vi "Teleop.vi"(10 "Match Info":T1={"Autonomous Elapsed Seconds"=0.0, "TeleOp Elapsed Seconds"=0.0, "Disabled Elapsed Seconds"=0.0, "Visited Autonomous"=FALSE, "Visited TeleOp"=FALSE, "Visited Disabled"=FALSE, "Autonomous Settings"={"Autonomous Style"=enum."Independent", "VI Refnum"=refnum}}, 11 "Call Context":T2) -> ()   [LabVIEW 2014]
doc: "This VI is called for each TeleOp packet received from the DS where the robot is not disabled. It is often used to read from the joysticks and update I/O or to update setpoints for timed control loops. It should complete and return within 20 milliseconds or it may miss DS packets."
uses:
  <vilib>/Rock Robotics/WPI/DriverStation/WPI_DriverStationDerivedRobotMode.ctl
  <vilib>/Rock Robotics/WPI/DriverStation/WPI_DriverStationMatch Info.ctl
  <vilib>/Rock Robotics/WPI/DriverStation/DriverStationLCD/WPI_DriverStationLCDLCDLine.ctl
  <vilib>/Rock Robotics/WPI/Joystick/WPI_JoystickGetSetRefNum.vi
  Robot Global Data.vi
  <vilib>/Rock Robotics/WPI/RobotDrive/WPI_RobotDriveGetSetRefNum.vi
  <vilib>/Rock Robotics/WPI/RobotDrive/WPI_RobotDriveArcadeDrive_Standard(NoSaturation).vi
  <vilib>/Rock Robotics/WPI/Solenoid/Deprecated/WPI_SolenoidSetBool.vi
panel:
  out "Numeric 1":dbl(slide) scale=0.0..100.0
  out "Boolean 2":bool
  out "Boolean 1":bool
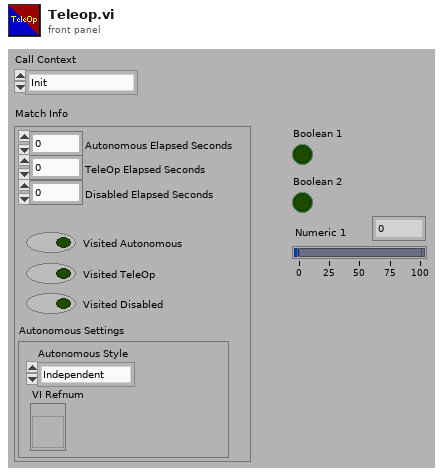
[diagram p1: front panel]
types:
  T1 = typedef "WPI_DriverStationMatch Info.ctl" = cluster{"Autonomous Elapsed Seconds":dbl, "TeleOp Elapsed Seconds":dbl, "Disabled Elapsed Seconds":dbl, "Visited Autonomous":bool, "Visited TeleOp":bool, "Visited Disabled":bool, "Autonomous Settings":cluster{"Autonomous Style":enum16{"Iterative", "Independent"}, "VI Refnum":refnum<vi>}}
  T2 = typedef "WPI_DriverStationDerivedRobotMode.ctl" = enum16{"Init", "Execute", "Stop"}
  T3 = typedef "WPI_DriverStationLCDLCDLine.ctl" = enum16{"Main - Line 1", "User - Line 2", "User - Line 3", "User - Line 4", "User - Line 5", "User - Line 6"}
  T4 = typedef "WPI_DigitalInputDevRef.ctl" = cluster{"DevStatus":errorcluster, "DIO Channel":T5, "Digital Module":T6}
  T5 = typedef "FPGA_DIOChannel.ctl" = enum8{"DIO 1", "DIO 2", "DIO 3", "DIO 4", "DIO 5", "DIO 6", "DIO 7", "DIO 8", "DIO 9", "DIO 10", "DIO 11", "DIO 12", "DIO 13", "DIO 14", "Invalid"}
  T6 = typedef "FPGA_TypedefDigitalModule.ctl" = enum16{"Digital Module 1", "Digital Module 2"}
  T7 = typedef "WPI_JoystickDevRef.ctl" = cluster{"Device":T8}
  T8 = typedef "WPI_JoystickDeviceEnum.ctl" = enum16{"USB 0", "USB 1", "USB 2", "USB 3", "USB 4", "USB 5"}
  T9 = cluster{"Button 1":bool, "Button 2":bool, "Button 3":bool, "Button 4":bool, "Button 5":bool, "Button 6":bool, "Button 7":bool, "Button 8":bool, "Button 9":bool, "Button 10":bool, "Button 11":bool, "Button 12":bool}
  T10 = cluster{"axis 1 (x)":dbl, "axis 2 (y)":dbl, "axis 3 (throttle)":dbl, "axis 4":dbl, "axis 5":dbl, "axis 6":dbl}
  T11 = typedef "WPI_MotorControlDeviceRef.ctl" = cluster{"DeviceStatus":errorcluster, "Type":enum16{"PWM", "CAN"}, "PWM":cluster{"Digital Module":T6, "PWM Channel":T12, "DeadBand":T13}, "CAN":cluster{"Device Number":u8, "Control Mode":T14, "Semaphore":T15, "Max Vout":dbl}, "Invert":bool, "TransformRef":T16, "InvTransformRef":T16}
  T12 = typedef "FPGA_DIOPWMChannel.ctl" = enum8{"PWM 1", "PWM 2", "PWM 3", "PWM 4", "PWM 5", "PWM 6", "PWM 7", "PWM 8", "PWM 9", "PWM 10", "Invalid"}
  T13 = typedef "WPI_PWMDeadband.ctl" = cluster{"Name":string, "maxPositivePwm":i32, "minPositivePwm":i32, "centerPwm":i32, "maxNegativePwm":i32, "minNegativePwm":i32, "angularRange":u16}
  T14 = typedef "WPI_CANJaguar_ControlMode.ctl" = enum8{"Percent VBus", "Current", "Speed", "Position", "Voltage"}
  T15 = typedef "Semaphore RefNum" = refnum<k1>
  T16 = typedef "WPI_PWMTransform_ConPane.ctl" = refnum<vi>
  T17 = typedef "WPI_SolenoidDevRef.ctl" = cluster{"DevStatus":errorcluster, "Solenoid Module":T18, "Forward Solenoid Channel":T19, "Reverse Solenoid Channel":T19}
  T18 = typedef "FPGA_TypedefSolenoidModule.ctl" = enum16{"Solenoid Module 1", "Solenoid Module 2"}
  T19 = typedef "WPI_SolenoidChannel.ctl" = enum8{"Solenoid 1", "Solenoid 2", "Solenoid 3", "Solenoid 4", "Solenoid 5", "Solenoid 6", "Solenoid 7", "Solenoid 8", "Invalid"}
  T20 = typedef "WPI_RobotDriveDevRef.ctl" = cluster{"DevStatus":errorcluster, "Motors[]":T11[], "Square Inputs":bool, "Max Output":dbl}
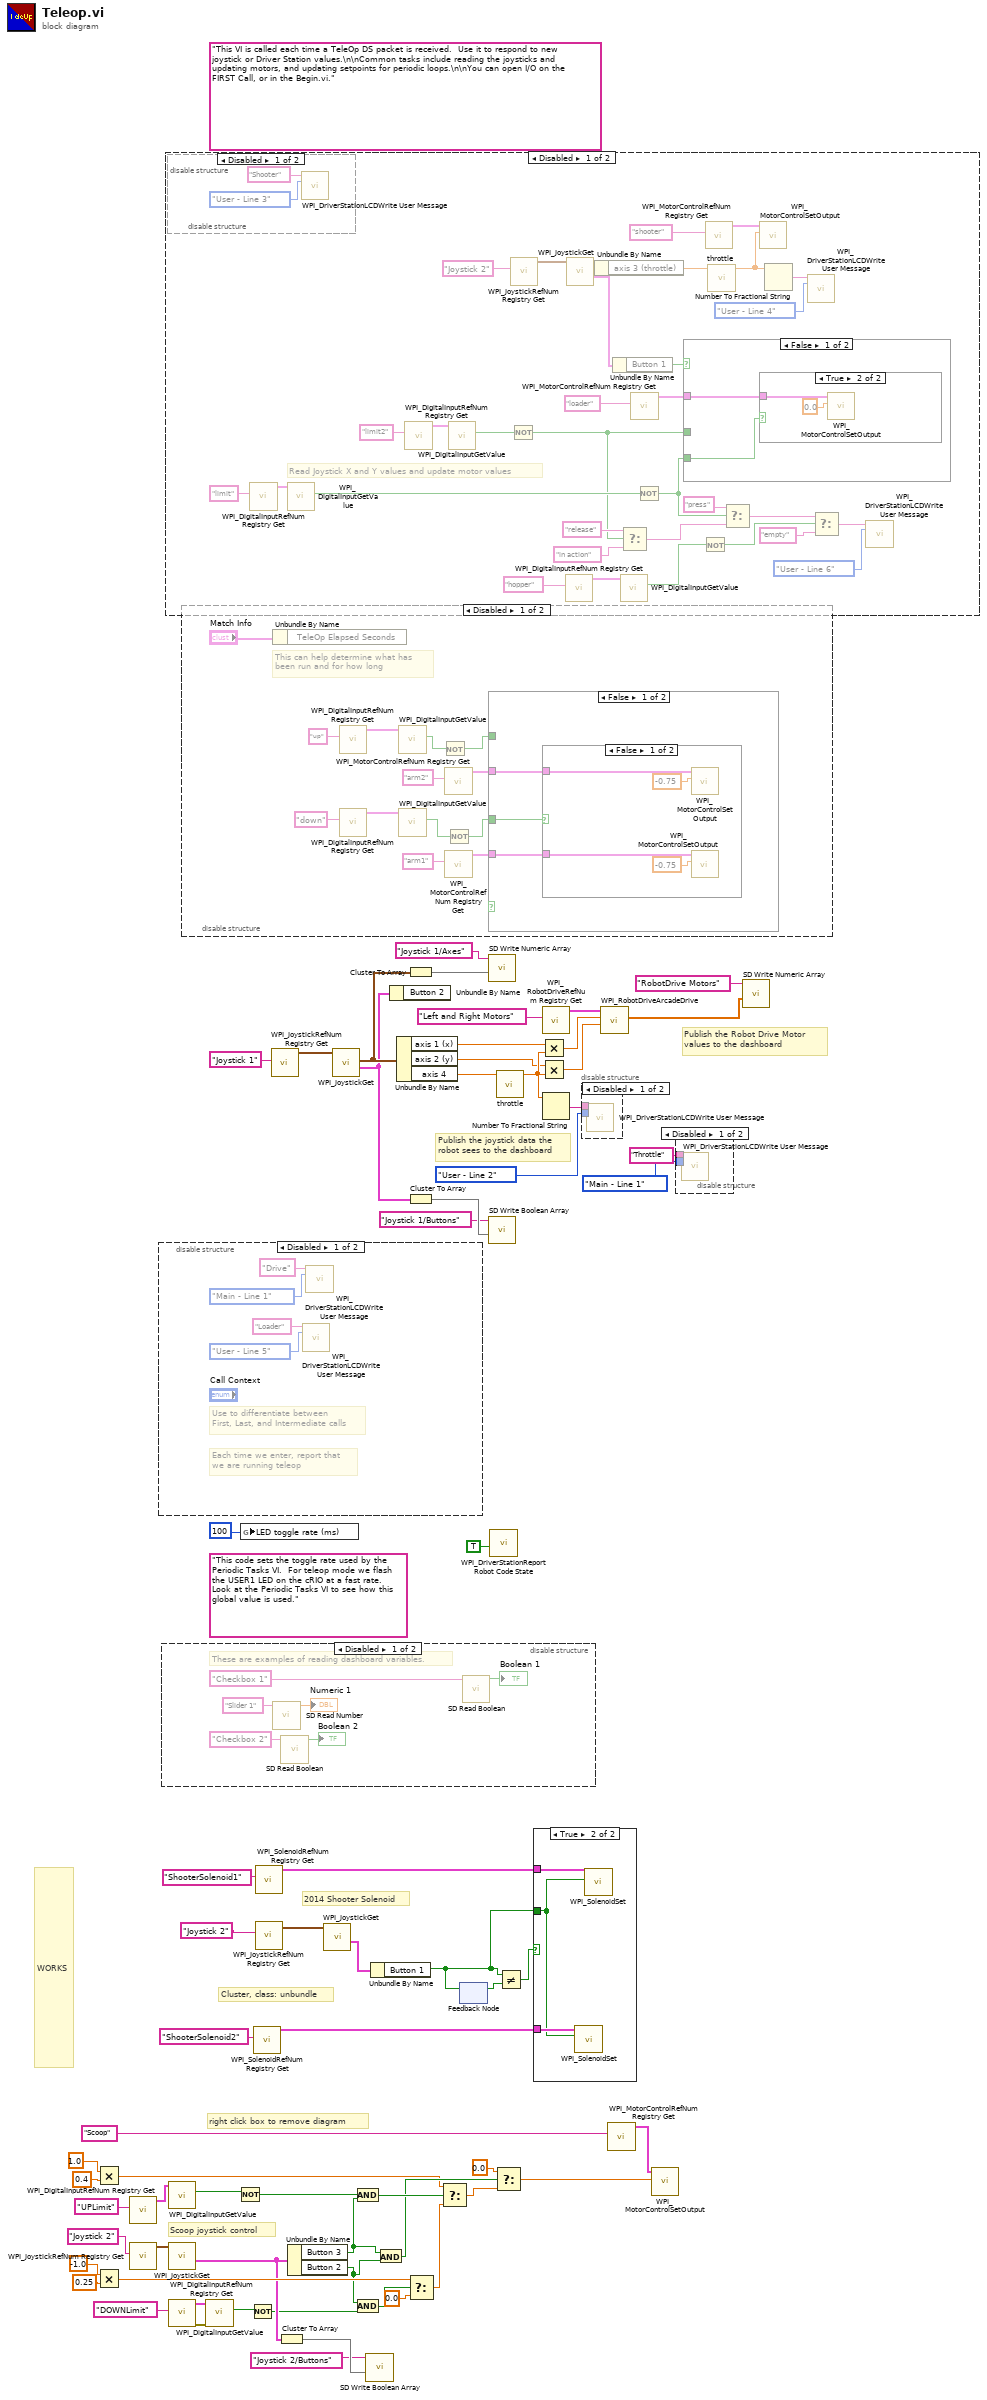
[diagram p0: block diagram]
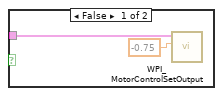
[diagram p4: hidden frame]
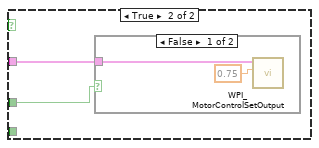
[diagram p5: hidden frame]
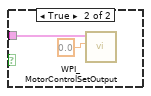
[diagram p6: hidden frame]
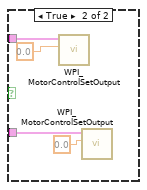
[diagram p12: hidden frame]
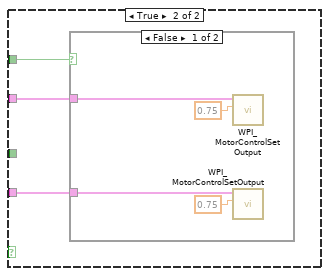
[diagram p13: hidden frame]
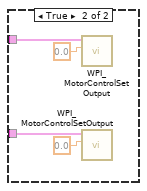
[diagram p14: hidden frame]
diagram:
  (unwired) "This code sets the toggle rate used by the Periodic Tasks VI.  For teleop mode we flash the USER1 LED on the cRIO at a fast rate.  Look at the Periodic Tasks VI to see how this global value is used."
  (unwired) "This VI is called each time a TeleOp DS packet is received.  Use it to respond to new joystick or Driver Station values.\n\nCommon tasks include reading the joysticks and updating motors, and updating setpoints for periodic loops.\n\nYou can open I/O on the FIRST Call, or in the Begin.vi."
  # "right click box to remove diagram"
  # "Scoop joystick control"
  # "WORKS"
  # "2014 Shooter Solenoid"
  # "Cluster, class: unbundle"
  # "Publish the Robot Drive Motor\nvalues to the dashboard"
  # "Publish the joystick data the\nrobot sees to the dashboard"
  n1 = Multiply(x=1.0, y=0.4) -> (x*y=w14:dbl)
  n2 = Multiply(x=-1.0, y=0.25) -> (x*y=w15:dbl)
  n3 = call <vilib>:"WPI_DigitalInputRefNum Registry Get.vi"("refnum name"="UPLimit") -> ("DigitalInputDevRef"=w29:T4)  [unwired: 9 in, 1 out]
  n4 = call <vilib>:"WPI_JoystickRefNum Registry Get.vi"("refnum name"="Joystick 2") -> ("JoystickDevRef"=w32:T7)  [unwired: 9 in, 1 out]
  n5 = disable-structure shown="Disabled" {
    frame Disabled {
      # "Each time we enter, report that\nwe are running teleop"
      # "Use to differentiate between\nFirst, Last, and Intermediate calls"
      n6 = call <vilib>:"WPI_DriverStationLCDWrite User Message.vi"("line text"="Loader", "line"=WPI_DriverStationLCDLCDLine."User - Line 5") -> ()  [unwired: 13 in, 1 out]
      n7 = call <vilib>:"WPI_DriverStationLCDWrite User Message.vi"("line text"="Drive", "line"=WPI_DriverStationLCDLCDLine."Main - Line 1") -> ()  [unwired: 13 in, 1 out]
    }
    frame Enabled {
    }
  }
  n8 = disable-structure shown="Disabled" {
    frame Disabled {
      # "These are examples of reading dashboard variables."
      n9 = call <vilib>:"SD Read Number.vi"("Name"="Slider 1" ("refnum name")) -> ("Numeric"=→"Numeric 1":dbl)  [unwired: 8 in, 2 out]
      n10 = call <vilib>:"SD Read Boolean.vi"("Name"="Checkbox 2" ("refnum name")) -> ("Boolean"=→"Boolean 2":bool)  [unwired: 8 in, 2 out]
      n11 = call <vilib>:"SD Read Boolean.vi"("Name"="Checkbox 1" ("refnum name")) -> ("Boolean"=→"Boolean 1":bool)  [unwired: 8 in, 2 out]
    }
    frame Enabled {
    }
  }
  n12 = disable-structure shown="Disabled" {
    frame Disabled {
      # "Read Joystick X and Y values and update motor values"
      n13 = disable-structure shown="Disabled" {
        frame Disabled {
          n14 = call <vilib>:"WPI_DriverStationLCDWrite User Message.vi"("line text"="Shooter", "line"=WPI_DriverStationLCDLCDLine."User - Line 3") -> ()  [unwired: 13 in, 1 out]
        }
        frame Enabled {
        }
      }
      n15 = call <vilib>:"WPI_DigitalInputRefNum Registry Get.vi"("refnum name"="limit") -> ("DigitalInputDevRef"=w106:T4)  [unwired: 9 in, 1 out]
      n16 = call <vilib>:"WPI_DigitalInputGetValue.vi"("DigitalInputDevRef"=w106) -> ("Value"=w100:bool)  [unwired: 8 in, 2 out]
      n17 = call <vilib>:"WPI_DigitalInputRefNum Registry Get.vi"("refnum name"="limit2") -> ("DigitalInputDevRef"=w102:T4)  [unwired: 9 in, 1 out]
      n18 = call <vilib>:"WPI_DigitalInputGetValue.vi"("DigitalInputDevRef"=w102) -> ("Value"=w101:bool)  [unwired: 8 in, 2 out]
      n19 = Not(x=w101) -> (.not. x?=w94:bool)
      n20 = call <vilib>:"WPI_JoystickRefNum Registry Get.vi"("refnum name"="Joystick 2") -> ("JoystickDevRef"=w92:T7)  [unwired: 1 in, 9 out]
      n21 = call <vilib>:"WPI_DigitalInputRefNum Registry Get.vi"("refnum name"="hopper") -> ("DigitalInputDevRef"=w82:T4)  [unwired: 9 in, 1 out]
      n22 = call <vilib>:"WPI_JoystickGet.vi"("JoystickDevRef"=w92) -> ("Buttons"=w89:T9, "Axes"=w90:T10)  [unwired: 1 in, 4 out]
      n23 = Unbundle By Name(w90) -> ("axis 3 (throttle)"=w88:dbl)
      n24 = Unbundle By Name(w89) -> ("Button 1"=w85:bool)
      n25 = call <vilib>:"WPI_DigitalInputGetValue.vi"("DigitalInputDevRef"=w82) -> ("Value"=w81:bool)  [unwired: 8 in, 2 out]
      n26 = Select(t="release", s=w94, f="in action") -> (s? t:f=w99:string)
      n27 = call <vilib>:"WPI_MotorControlRefNum Registry Get.vi"("refnum name"="loader") -> ("MotorControlDevRef"=w93:T11)  [unwired: 9 in, 1 out]
      n28 = Not(x=w100) -> (.not. x?=w95:bool)
      n29 = case shown="False" w85 {
        tunnel: w93 -> [w110 w116]
        tunnel: w94 -> [_ w117]
        tunnel: w95 -> [w111 _]
        frame False {
          n30 = case shown="True" w111 {
            tunnel: w110 -> [w112 w114]
            frame False {
              n31 = call <vilib>:"WPI_MotorControlSetOutput.vi"("Output"=-0.75, "MotorControlDevRef"=w112) -> ()  [unwired: 7 in, 3 out]
            }
            frame True {
              n32 = call <vilib>:"WPI_MotorControlSetOutput.vi"("Output"=0.0, "MotorControlDevRef"=w114) -> ()  [unwired: 7 in, 3 out]
            }
          }
        }
        frame True {
          n33 = case shown="False" w117 {
            tunnel: w116 -> [w119 w121]
            frame False {
              n34 = call <vilib>:"WPI_MotorControlSetOutput.vi"("Output"=0.75, "MotorControlDevRef"=w119) -> ()  [unwired: 7 in, 3 out]
            }
            frame True {
              n35 = call <vilib>:"WPI_MotorControlSetOutput.vi"("Output"=0.0, "MotorControlDevRef"=w121) -> ()  [unwired: 7 in, 3 out]
            }
          }
        }
      }
      n36 = Not(x=w81) -> (.not. x?=w78:bool)
      n37 = call <vilib>:"WPI_MotorControlRefNum Registry Get.vi"("refnum name"="shooter") -> ("MotorControlDevRef"=w109:T11)  [unwired: 9 in, 1 out]
      n38 = call "throttle.vi"("x"=w88) -> ("x/y"=w84:dbl)  [unwired: 10 in]
      n39 = Select(t="press", s=w95, f=w99) -> (s? t:f=w80:string)
      n40 = call <vilib>:"WPI_MotorControlSetOutput.vi"("Output"=w84, "MotorControlDevRef"=w109) -> ()  [unwired: 7 in, 3 out]
      n41 = Number To Fractional String(number=w84) -> (F-format string=w87:string)  [unwired: 3 in]
      n42 = call <vilib>:"WPI_DriverStationLCDWrite User Message.vi"("line text"=w87, "line"=WPI_DriverStationLCDLCDLine."User - Line 4") -> ()  [unwired: 13 in, 1 out]
      n43 = Select(t=w80, s=w78, f="empty") -> (s? t:f=w79:string)
      n44 = call <vilib>:"WPI_DriverStationLCDWrite User Message.vi"("line text"=w79, "line"=WPI_DriverStationLCDLCDLine."User - Line 6") -> ()  [unwired: 13 in, 1 out]
    }
    frame Enabled {
    }
  }
  n45 = call <vilib>:"WPI_DigitalInputGetValue.vi"("DigitalInputDevRef"=w29) -> ("Value"=w5:bool)  [unwired: 8 in, 2 out]
  n46 = call <vilib>:"WPI_JoystickGet.vi"("JoystickDevRef"=w32) -> ("Buttons"=w8:T9)  [unwired: 4 in, 2 out]
  n47 = call <vilib>:"WPI_DigitalInputRefNum Registry Get.vi"("refnum name"="DOWNLimit") -> ("error out"=w31:errorcluster, "DigitalInputDevRef"=w30:T4)  [unwired: 9 in]
  n48 = disable-structure shown="Disabled" {
    frame Disabled {
      # "This can help determine what has\nbeen run and for how long"
      n49 = Unbundle By Name("Match Info") -> ()  [unwired: 1 out]
      n50 = call <vilib>:"WPI_DigitalInputRefNum Registry Get.vi"("refnum name"="up") -> ("DigitalInputDevRef"=w135:T4)  [unwired: 9 in, 1 out]
      n51 = call <vilib>:"WPI_DigitalInputRefNum Registry Get.vi"("refnum name"="down") -> ("DigitalInputDevRef"=w134:T4)  [unwired: 9 in, 1 out]
      n52 = call <vilib>:"WPI_DigitalInputGetValue.vi"("DigitalInputDevRef"=w135) -> ("Value"=w127:bool)  [unwired: 8 in, 2 out]
      n53 = call <vilib>:"WPI_DigitalInputGetValue.vi"("DigitalInputDevRef"=w134) -> ("Value"=w125:bool)  [unwired: 8 in, 2 out]
      n54 = Not(x=w127) -> (.not. x?=w126:bool)
      n55 = call <vilib>:"WPI_MotorControlRefNum Registry Get.vi"("refnum name"="arm2") -> ("MotorControlDevRef"=w130:T11)  [unwired: 9 in, 1 out]
      n56 = call <vilib>:"WPI_MotorControlRefNum Registry Get.vi"("refnum name"="arm1") -> ("MotorControlDevRef"=w131:T11)  [unwired: 9 in, 1 out]
      n57 = Not(x=w125) -> (.not. x?=w124:bool)
      n58 = case shown="False" {
        selector: _ -> [_ _]
        tunnel: w126 -> [_ w150]
        tunnel: w124 -> [w139 _]
        tunnel: w131 -> [w138 w149]
        tunnel: w130 -> [w137 w148]
        frame False {
          n59 = case shown="False" w139 {
            tunnel: w138 -> [w141 w146]
            tunnel: w137 -> [w140 w145]
            frame False {
              n60 = call <vilib>:"WPI_MotorControlSetOutput.vi"("Output"=-0.75, "MotorControlDevRef"=w140) -> ()  [unwired: 7 in, 3 out]
              n61 = call <vilib>:"WPI_MotorControlSetOutput.vi"("Output"=-0.75, "MotorControlDevRef"=w141) -> ()  [unwired: 7 in, 3 out]
            }
            frame True {
              n62 = call <vilib>:"WPI_MotorControlSetOutput.vi"("Output"=0.0, "MotorControlDevRef"=w145) -> ()  [unwired: 7 in, 3 out]
              n63 = call <vilib>:"WPI_MotorControlSetOutput.vi"("Output"=0.0, "MotorControlDevRef"=w146) -> ()  [unwired: 7 in, 3 out]
            }
          }
        }
        frame True {
          n64 = case shown="False" w150 {
            tunnel: w149 -> [w152 w156]
            tunnel: w148 -> [w151 w155]
            frame False {
              n65 = call <vilib>:"WPI_MotorControlSetOutput.vi"("Output"=0.75, "MotorControlDevRef"=w151) -> ()  [unwired: 7 in, 3 out]
              n66 = call <vilib>:"WPI_MotorControlSetOutput.vi"("Output"=0.75, "MotorControlDevRef"=w152) -> ()  [unwired: 7 in, 3 out]
            }
            frame True {
              n67 = call <vilib>:"WPI_MotorControlSetOutput.vi"("Output"=0.0, "MotorControlDevRef"=w155) -> ()  [unwired: 7 in, 3 out]
              n68 = call <vilib>:"WPI_MotorControlSetOutput.vi"("Output"=0.0, "MotorControlDevRef"=w156) -> ()  [unwired: 7 in, 3 out]
            }
          }
        }
      }
    }
    frame Enabled {
    }
  }
  n69 = call <vilib>:"WPI_DigitalInputGetValue.vi"("error in (no error)"=w31, "DigitalInputDevRef"=w30) -> ("Value"=w7:bool)  [unwired: 7 in, 2 out]
  n70 = Not(x=w5) -> (.not. x?=w4:bool)
  n71 = global write "Robot Global Data.vi" "LED toggle rate (ms)"(u32 100 ("LED ms toggle rate")) -> ()
  n72 = Not(x=w7) -> (.not. x?=w6:bool)
  n73 = call <vilib>:"WPI_SolenoidRefNum Registry Get.vi"("refnum name"="ShooterSolenoid2") -> ("SolenoidDevRef"=w39:T17)  [unwired: 9 in, 1 out]
  n74 = call <vilib>:"WPI_SolenoidRefNum Registry Get.vi"("refnum name"="ShooterSolenoid1") -> ("SolenoidDevRef"=w44:T17)  [unwired: 9 in, 1 out]
  n75 = call <vilib>:"WPI_JoystickRefNum Registry Get.vi"("refnum name"="Joystick 2") -> ("JoystickDevRef"=w43:T7)  [unwired: 9 in, 1 out]
  n76 = call <vilib>:"WPI_JoystickRefNum Registry Get.vi"("refnum name"="Joystick 1") -> ("JoystickDevRef"=w64:T7)  [unwired: 1 in, 9 out]
  n77 = Cluster To Array(cluster=w8) -> (array=w10:bool[])
  n78 = Unbundle By Name(w8) -> ("Button 3"=w12:bool, "Button 2"=w11:bool)
  n79 = call <vilib>:"WPI_JoystickGet.vi"("JoystickDevRef"=w43) -> ("Buttons"=w41:T9)  [unwired: 4 in, 2 out]
  n80 = call <vilib>:"WPI_JoystickGet.vi"("JoystickDevRef"=w64) -> ("Buttons"=w46:T9, "Axes"=w60:T10)  [unwired: 1 in, 4 out]
  n81 = And(x=w4, y=w12) -> (x .and. y?=w26:bool)
  n82 = And(x=w11, y=w6) -> (x .and. y?=w25:bool)
  n83 = call <vilib>:"SD Write Boolean Array.vi"("Boolean Array"=w10, "Name"="Joystick 2/Buttons") -> ()  [unwired: 8 in, 2 out]
  n84 = Unbundle By Name(w41) -> ("Button 1"=w36:bool)
  n85 = And(x=w12, y=w11) -> (x .and. y?=w21:bool)
  n86 = Unbundle By Name(w46) -> ()  [unwired: 1 out]
  n87 = Unbundle By Name(w60) -> ("axis 1 (x)"=w53:dbl, "axis 2 (y)"=w47:dbl, "axis 4"=w55:dbl)
  n88 = Cluster To Array(cluster=w60) -> (array=w59:dbl[])
  n89 = Cluster To Array(cluster=w46) -> (array=w62:bool[])
  n90 = Select(t=w15, s=w25, f=0.0) -> (s? t:f=w19:dbl)
  n91 = Select(t=w14, s=w26, f=w19) -> (s? t:f=w23:dbl)
  n92 = feedback-in #1(w36) -> ()
  n93 = feedback #1() -> (w37:bool)  [unwired: 1 in]
  n94 = call <vilib>:"SD Write Numeric Array.vi"("Numeric Array"=w59, "Name"="Joystick 1/Axes") -> ()  [unwired: 8 in, 2 out]
  n95 = call <vilib>:"SD Write Boolean Array.vi"("Boolean Array"=w62, "Name"="Joystick 1/Buttons") -> ()  [unwired: 8 in, 2 out]
  n96 = call <vilib>:"WPI_DriverStationReport Robot Code State.vi"("TeleOp"=TRUE ("Autonomous")) -> ()  [unwired: 10 in, 1 out]
  n97 = Select(t=0.0, s=w21, f=w23) -> (s? t:f=w13:dbl)
  n98 = call "throttle.vi"("x"=w55) -> ("x/y"=w50:dbl)  [unwired: 10 in]
  n99 = Not Equal?(x=w36, y=w37) -> (x != y?=w38:bool)
  n100 = case shown="True" w38 {
    tunnel: w44 -> [_ w161]
    tunnel: w39 -> [_ w160]
    tunnel: w36 -> [_ w159]
    frame False {
    }
    frame True {
      n101 = call-poly <vilib>:"WPI_SolenoidSet.vi"("Value"=w159, "SolenoidDevRef"=w160) -> ()  [unwired: 8 in, 2 out]
      n102 = call-poly <vilib>:"WPI_SolenoidSet.vi"("Value"=w159, "SolenoidDevRef"=w161) -> ()  [unwired: 8 in, 2 out]
    }
  }
  n103 = Multiply(x=w53, y=w50) -> (x*y=w52:dbl)
  n104 = Multiply(x=w47, y=w50) -> (x*y=w54:dbl)
  n105 = call <vilib>:"WPI_RobotDriveRefNum Registry Get.vi"("refnum name"="Left and Right Motors") -> ("RobotDriveDevRef"=w48:T20)  [unwired: 1 in, 9 out]
  n106 = Number To Fractional String(number=w50) -> (F-format string=w51:string)  [unwired: 3 in]
  n107 = disable-structure shown="Disabled" {
    disable-tunnel: w51 -> [w163 _]
    disable-tunnel: WPI_DriverStationLCDLCDLine."User - Line 2" ("line") -> [w162 _]
    frame Disabled {
      n108 = call <vilib>:"WPI_DriverStationLCDWrite User Message.vi"("line text"=w163, "line"=w162) -> ()  [unwired: 13 in, 1 out]
    }
    frame Enabled {
    }
  }
  n109 = call-poly <vilib>:"WPI_RobotDriveArcadeDrive.vi"("Y axis value"=w54, "X axis value"=w52, "RobotDriveDevRef"=w48) -> ("Motor Values"=w56:dbl[])  [unwired: 6 in, 2 out]
  n110 = call <vilib>:"WPI_MotorControlRefNum Registry Get.vi"("refnum name"="Scoop") -> ("MotorControlDevRef"=w34:T11)  [unwired: 9 in, 1 out]
  n111 = call <vilib>:"WPI_MotorControlSetOutput.vi"("Output"=w13, "MotorControlDevRef"=w34) -> ()  [unwired: 7 in, 3 out]
  n112 = disable-structure shown="Disabled" {
    disable-tunnel: "Throttle" ("line text") -> [w165 _]
    disable-tunnel: WPI_DriverStationLCDLCDLine."Main - Line 1" ("line") -> [w164 _]
    frame Disabled {
      n113 = call <vilib>:"WPI_DriverStationLCDWrite User Message.vi"("line text"=w165, "line"=w164) -> ()  [unwired: 13 in, 1 out]
    }
    frame Enabled {
    }
  }
  n114 = call <vilib>:"SD Write Numeric Array.vi"("Numeric Array"=w56, "Name"="RobotDrive Motors") -> ()  [unwired: 8 in, 2 out]
